vi "NavX Zero Heading.vi"(8 "error in":errorcluster, 11 "Default Heading":dbl=-400.0) -> (0 "error out":errorcluster)   [LabVIEW 2015]
uses:
  Support/Global Objects.vi
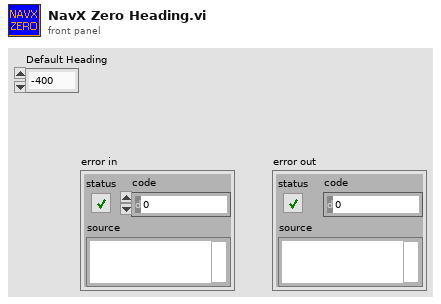
[diagram p1: front panel]
types:
  T1 = typedef "NaxX Info.ctl" = cluster{"navX Device":T2, "Current Yaw":dbl, "Active":bool}
  T2 = typedef "navX Library v2.lvlib/Z900_navX_DeviceTypeDef.ctl" = cluster{"Interface":cluster{"Protocol":T3, "Update Rate (4Hz-60Hz)":u8, "navX Open TypeDef":variant}, "Notify Packet":refnum<notifier>, "Loop VI Refnum":refnum<vi>, "Ready to Close Occurrence Refnum":refnum<k4>}
  T3 = typedef "navX Library v2.lvlib/Z900_navX_ProtocolTypeDef.ctl" = enum16{"SERIAL", "I2C", "SPI"}
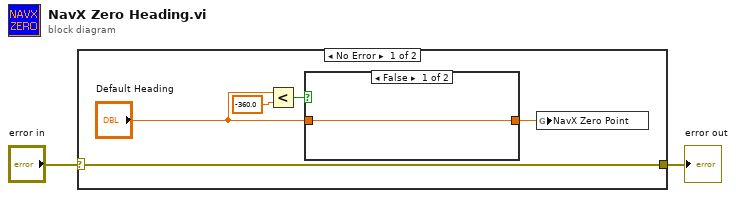
[diagram p0: block diagram]
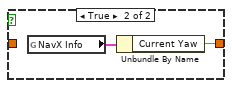
[diagram p2: hidden frame]
diagram:
  n1 = case shown="No Error" "error in" {
    selector: "error in" -> [w7 w11]
    tunnel: [w7 w11] -> w1
    frame No Error {
      n2 = Less?(x="Default Heading", y=-360.0) -> (x < y?=w5:bool)
      n3 = case shown="False" w5 {
        tunnel: [w8 w9] -> w4
        tunnel: "Default Heading" -> [w8 _]
        frame False {
        }
        frame True {
          n4 = global read "Global Objects.vi" "NavX Info"() -> (w10:T1)
          n5 = Unbundle By Name(w10) -> ("Current Yaw"=w9:dbl)
        }
      }
      n6 = global write "Global Objects.vi" "NavX Zero Point"(w4) -> ()
    }
    frame Error {
    }
  }
  "error out" <- w1
